vi "rad_Reboot (IP) Wrapper.vi"(5 "Password":string, 8 "error in (no error)":errorcluster, 10 "wait for restart? (F)":bool, 11 "Target settings in":T1={"Hostname"="", "Serial number"="", "Product name"="", "Product code"=0, "System status"="", "Credential type"=enum."None/Unlocked", "User added?"=FALSE, "Primary NIC"={"MAC address"="", "IP Address Request Mode"=2, "IP address"="", "Subnet mask"="", "Gateway"="", "DNS server"=""}} {"Primary NIC"."IP Address Request Mode" items=["Static"=1, "DHCP/Link-Local"=2, "Link-Local Only"=4, "DHCP Only"=8]}) -> (0 "error out":errorcluster, 3 "Target settings out":T1={"Hostname"="", "Serial number"="", "Product name"="", "Product code"=0, "System status"="", "Credential type"=enum."None/Unlocked", "User added?"=FALSE, "Primary NIC"={"MAC address"="", "IP Address Request Mode"=2, "IP address"="", "Subnet mask"="", "Gateway"="", "DNS server"=""}} {"Primary NIC"."IP Address Request Mode" items=["Static"=1, "DHCP/Link-Local"=2, "Link-Local Only"=4, "DHCP Only"=8]})   [LabVIEW 2020]
uses:
  <vilib>/nisyscfg/nisyscfg.lvlib
  <vilib>/nisyscfg/Close (System).vi
  Targets/TypeDefs/rad_Target Information.ctl
  Targets/TypeDefs/rad_Target Network Settings.ctl
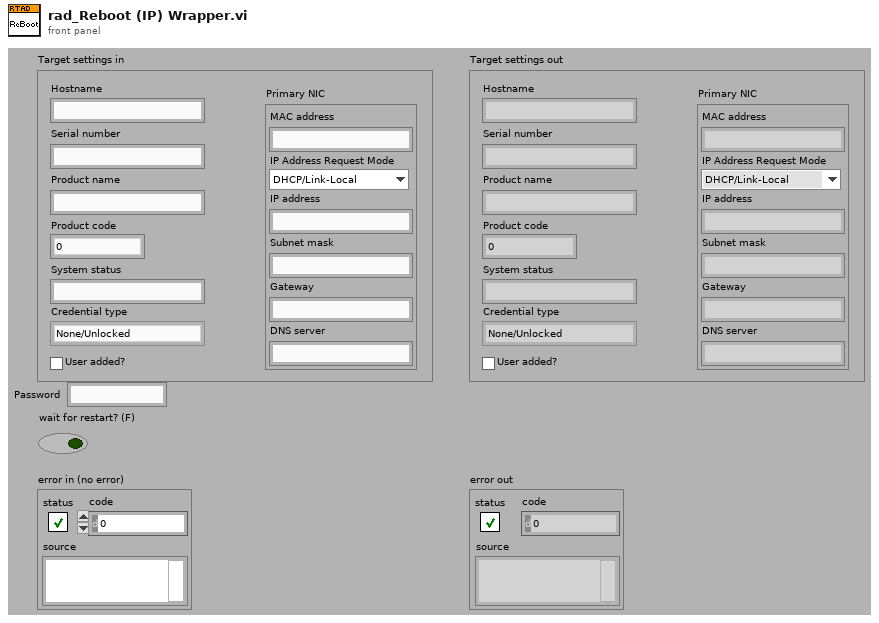
[diagram p1: front panel]
types:
  T1 = typedef "rad_Target Information.ctl" = cluster{"Hostname":string, "Serial number":string, "Product name":string, "Product code":i32, "System status":string, "Credential type":enum16{"None/Unlocked", "FTP Password", "NIAuth Credentials"}, "User added?":bool, "Primary NIC":T2}
  T2 = typedef "rad_Target Network Settings.ctl" = cluster{"MAC address":string, "IP Address Request Mode":i32, "IP address":string, "Subnet mask":string, "Gateway":string, "DNS server":string}
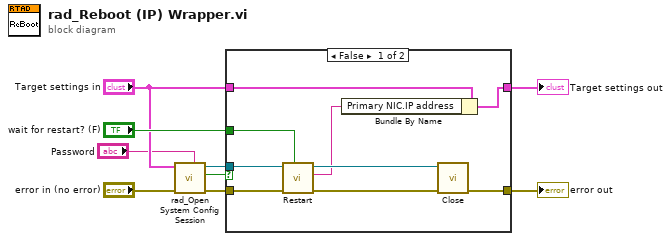
[diagram p0: block diagram]
diagram:
  n1 = call "rad_Open System Config Session.vi"("Password"="Password", "error in (no error)"="error in (no error)", "Target settings"="Target settings in") -> ("error out"=w4:errorcluster, "Cancelled"=w6:bool, "Session out"=w5:refnum<k21>)  [unwired: 5 in, 1 out]
  n2 = case shown="False" w6 {
    tunnel: "wait for restart? (F)" -> [w18 _]
    tunnel: [w13 w20] -> w7
    tunnel: w5 -> [w17 _]
    tunnel: w4 -> [w16 w20]
    tunnel: "Target settings in" -> [w12 w19]
    tunnel: [w11 w19] -> w2
    frame False {
      n3 = call <vilib>:"Restart.vi"("Wait Until Complete (T)"=w18, "error in (no error)"=w16, "Session in"=w17) -> ("error out"=w14:errorcluster, "New IP Address"=w10:string, "Session out"=w15:refnum<k21>)  [unwired: 6 in]
      n4 = Bundle By Name(cluster=w12, "Primary NIC.IP address"=w10) -> (w11:T1)
      n5 = call-poly <vilib>:"Close.vi"("error in (no error)"=w14, "Session in"=w15) -> ("error out"=w13:errorcluster)  [unwired: 9 in]
    }
    frame True {
    }
  }
  "error out" <- w7
  "Target settings out" <- w2
